vi "clamp_vals_array.vi"(8 "Min Val":dbl, 10 "Input Array":dbl[](array[numeric]), 11 "Max Val":dbl) -> (2 "Output Array":dbl[](array[numeric]))   [LabVIEW 2024]
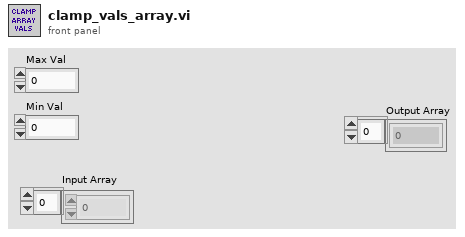
[diagram p1: front panel]
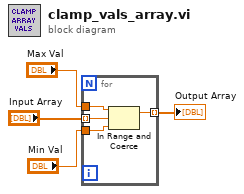
[diagram p0: block diagram]
diagram:
  n1 = for {
    tunnel: "Min Val" -> [w8]
    tunnel: "Max Val" -> [w7]
    tunnel: "Input Array" -> [w6] mode=indexing
    tunnel: [w5] -> w1 mode=indexing
    n2 = In Range and Coerce(upper limit=w7, x=w6, lower limit=w8) -> (coerced(x)=w5:dbl)  [unwired: 1 out]
  }
  "Output Array" <- w1
